vi "fakeScan.vi"() -> ()   [LabVIEW 2010]
uses:
  line_info.ctl
panel:
  out "line":T1
  out "size(s)":i32
  in  "CH1":bool=TRUE
  in  "CH0":bool=TRUE
  in  "xyz order":bool
  out "sort stats":T2
  out "assemble stats":T3
  in  "spilt ff/fb":bool
  out "lines":i32
  out "error out":errorcluster
  out "timed out?":bool
  out "XY view":T4(plugin-control)
  out "YZ view":T4(plugin-control)
  out "XZ view":T4(plugin-control)
  in  "scan specification":T5={"x amplitude"=100, "x resolution (pixels)"=30, "x offset fly-forward (iterations)"=57, "x offset fly-back (iterations)"=115, "y resolution (nr. of lines)"=79, "y step size"=41, "iterations per pixel"=5, "number of frames"=120, "y offset (pixels)"=0, "number of y-brake lines  (before y-fly-back)"=0, "number y-brake lines (after y-fly-back)"=30, "number of y-fly-back steps"=0, "lines per z step"=1, "number of z/intensity tuples"=342, "number of repetitions (volumes or planes)"=2, "z step size derived"=27, "choose the beginning of z scan"=FALSE, "number of frames (settings)"=120, "FPGA trajectory?"=TRUE, "Pockels cell voltage (bits)"=0, "Vy min(bits)"=-1638, "Vz min(bits)"=-1638}
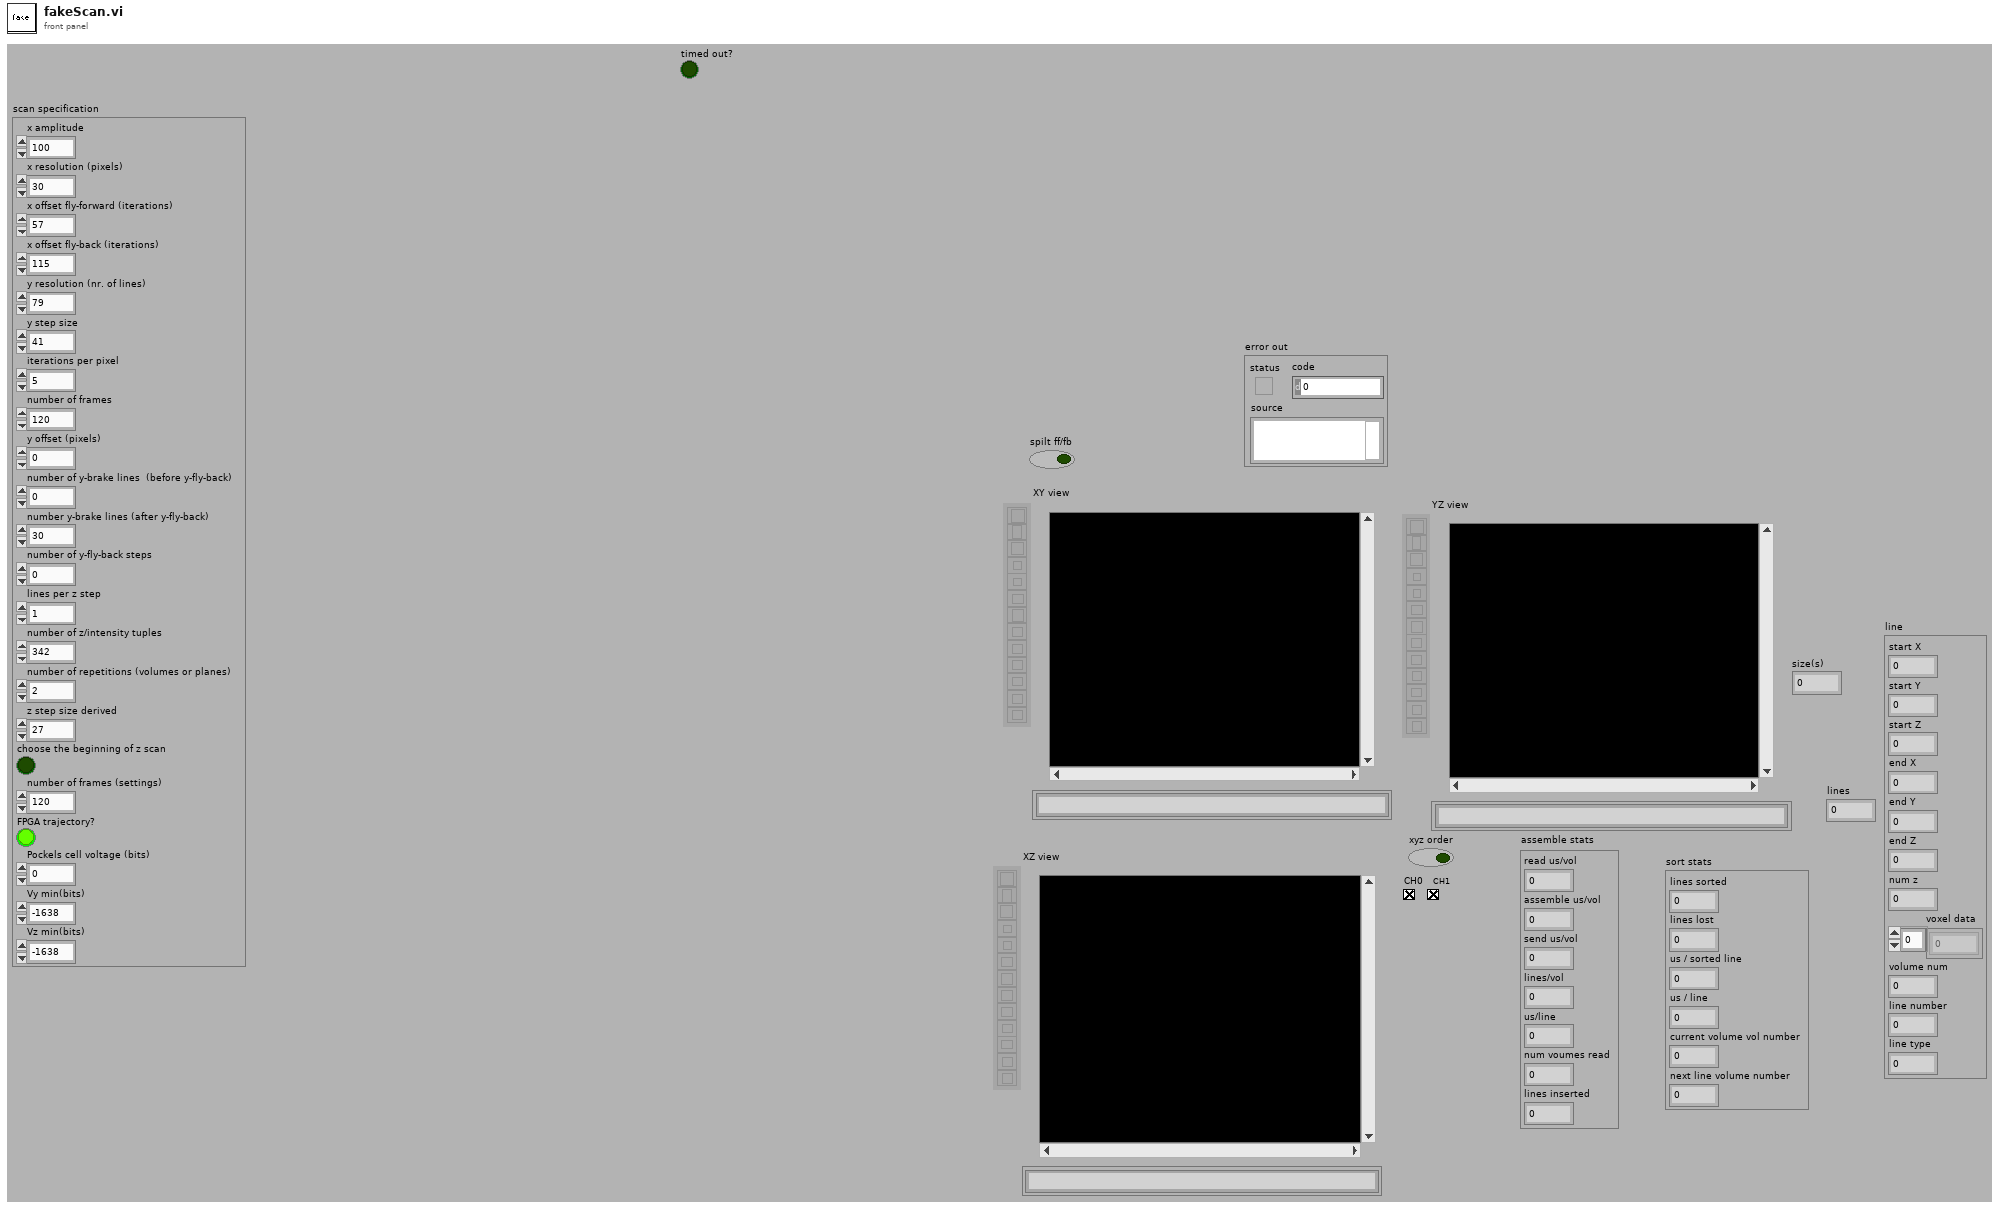
[diagram p1: front panel]
types:
  T1 = typedef "line_info.ctl" = cluster{"start X":i16, "start Y":i16, "start Z":i16, "end X":i16, "end Y":i16, "end Z":i16, "num z":u8, "voxel data":u32[], "volume num":u32, "line number":u16, "line type":u16}
  T2 = cluster{"lines sorted":i32, "lines lost":i32, "us / sorted line":dbl, "us / line":dbl, "current volume vol number":u32, "next line volume number":u32}
  T3 = cluster{"read us/vol":dbl, "assemble us/vol":dbl, "send us/vol":dbl, "lines/vol":dbl, "us/line":dbl, "num voumes read":u32, "lines inserted":i32}
  T4 = typedef "IMAQ Image.ctl" = refnum<image>
  T5 = cluster{"x amplitude":u16, "x resolution (pixels)":u16, "x offset fly-forward (iterations)":u16, "x offset fly-back (iterations)":u16, "y resolution (nr. of lines)":u16, "y step size":u16, "iterations per pixel":u16, "number of frames":i32, "y offset (pixels)":u16, "number of y-brake lines  (before y-fly-back)":u16, "number y-brake lines (after y-fly-back)":u16, "number of y-fly-back steps":u16, "lines per z step":u16, "number of z/intensity tuples":u16, "number of repetitions (volumes or planes)":i32, "z step size derived":u16, "choose the beginning of z scan":bool, "number of frames (settings)":i32, "FPGA trajectory?":bool, "Pockels cell voltage (bits)":i16, "Vy min(bits)":i16, "Vz min(bits)":i16}
  T6 = typedef "Image Type" = u32
  T7 = typedef "internal_queues.ctl" = cluster{"volumeQueue":refnum<queue>, "linesWithoutDataQueue":refnum<queue>, "lineQueue":refnum<queue>, "volumesWithLinesQueue":refnum<queue>, "kalmanQueue":refnum<queue>, "completedVolumeQueue":refnum<queue>, "displayVolumeQueue":refnum<queue>, "scanLocationsQueue":refnum<queue>, "kalmanToDisplayPanel":refnum<queue>, "focalPositionQueue":refnum<queue>, "spotPositionsToImagePanel":refnum<queue>}
  T8 = cluster{"min x":i16, "deltaX":dbl, "num x":u32, "max x":i16, "min y":i16, "deltaY":dbl, "num y":u32, "max y":i16, "num z":u32, "num voxels":u32, "voxels read":u32, "volume num":u32}
  T9 = cluster{"lines sorted":i32, "lines lost":i32, "us / sorted line":dbl, "us / line":dbl, "current volume vol number":u32, "next line volume number":u32, "volume rate(Hz)":dbl}
  T10 = cluster{"ch0 volume":u32[][][], "ch1 volume":u32[][][], "ff 0+1":u32[][][], "fb 0+1":u32[][][]}
  T11 = cluster{"New Image":T4, "New Image":T4, "New Image":T4}
  T12 = cluster{"Image Dst Out":T4, "Image Dst Out":T4, "Image Dst Out":T4}
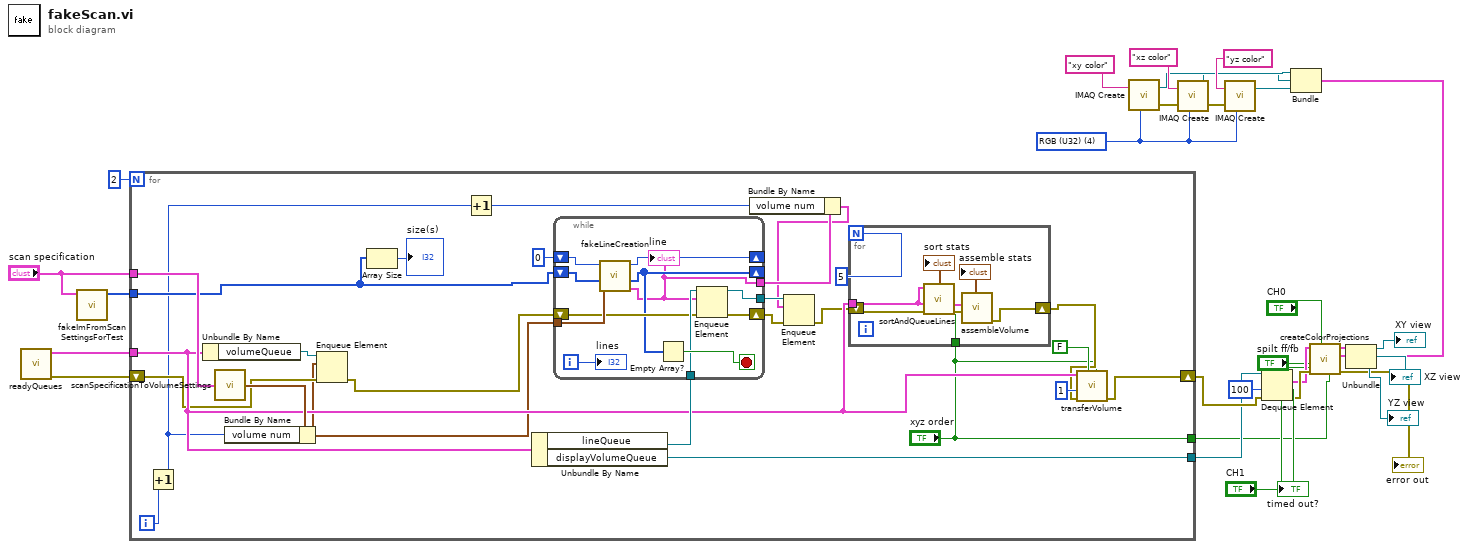
[diagram p0: block diagram]
diagram:
  w17 = T6 4 items=["Grayscale (U8)", "Grayscale (I16)", "Grayscale (SGL)", "Complex (CSG)", "RGB (U32)", "HSL (U32)", "RGB (U64)", "Grayscale (U16)"] ("Image Type")
  n1 = call "readyQueues.vi"() -> ("error out"=w8:errorcluster, "Queues"=w30:T7)  [unwired: 10 in]
  n2 = call "fakeImFromScanSettingsForTest.vi"("scan specification"="scan specification") -> ("fake 2 ch im"=w5:u32[])  [unwired: 10 in]
  n3 = for {
    N: 2 -> [_]
    tunnel: "scan specification" -> [w56]
    tunnel: w30 -> [w51]
    tunnel: [w47] -> w14
    shift-right: [w48] -> w15
    shift-left: w8 -> [w45]
    tunnel: w5 -> [w40]
    tunnel: ["xyz order"] -> w1
    i -> [w42]
    n4 = Increment(x=w42) -> (x+1=w33:i32)
    n5 = Unbundle By Name(w51) -> ("volumeQueue"=w36:refnum<queue>)
    n6 = call "scanSpecificationToVolumeSettings.vi"("scan specification"=w56) -> ("volume info"=w55:T8)
    n7 = Bundle By Name(cluster=w55, "volume num"=w33) -> (w43:T8)
    n8 = Enqueue Element(queue=w36, element=w43, error in (no error)=w45) -> (error out=w44:errorcluster)  [unwired: 1 in, 2 out]
    n9 = Array Size(array=w40) -> (size(s)=→"size(s)":i32)
    n10 = Increment(x=w33) -> (x+1=w32:i32)
    n11 = Unbundle By Name(w51) -> ("lineQueue"=w53:refnum<queue>, "displayVolumeQueue"=w47:refnum<queue>)
    n12 = while {
      tunnel: w43 -> [w75]
      shift-right: [w66] -> _
      shift-left: w40 -> [w67]
      shift-right: [w73] -> _
      shift-left: u32 0 ("voxel number out") -> [w72]
      tunnel: w53 -> [w71]
      shift-right: [w70] -> w38
      shift-left: w44 -> [w69]
      tunnel: [w65] -> w34
      tunnel: [w64] -> w35
      i -> [w68]
      stop <- w74 stop-if-true
      n13 = call "fakeLineCreation.vi"("volume info"=w75, "data stream in"=w67, "voxel number"=w72) -> ("line"=w65:T1, "data stream out"=w66:u32[], "voxel number out"=w73:u32)  [unwired: 6 in]
      "line" <- w65
      n14 = Empty Array?(array=w66) -> (empty?=w74:bool)
      n15 = Enqueue Element(queue=w71, element=w65, error in (no error)=w69) -> (queue out=w64:refnum<queue>, error out=w70:errorcluster)  [unwired: 1 in, 1 out]
      "lines" <- w68
    }
    n16 = Bundle By Name(cluster=w34, "volume num"=w32) -> (w31:T1)
    n17 = Enqueue Element(queue=w35, element=w31, error in (no error)=w38) -> (error out=w37:errorcluster)  [unwired: 1 in, 2 out]
    n18 = for {
      N: 5 -> [_]
      tunnel: w51 -> [w59]
      shift-right: [w63] -> w49
      shift-left: w37 -> [w61]
      tunnel: "xyz order" -> [w57]
      n19 = call "sortAndQueueLines.vi"("error in (no error)"=w61, "Queues"=w59) -> ("error out"=w60:errorcluster, "stats"=→"sort stats":T9)  [unwired: 6 in, 2 out]
      n20 = call "assembleVolume.vi"("error in (no error)"=w60, "xyz order"=w57, "Queues"=w59) -> ("error out"=w63:errorcluster, "status"=→"assemble stats":T3)  [unwired: 6 in, 1 out]
    }
    n21 = call "transferVolume.vi"("xyz order"="xyz order", "write to network stream"=FALSE, "error in (no error)"=w49, "num vol to sum"=u32 1, "Queues"=w51) -> ("error out"=w48:errorcluster)  [unwired: 1 in, 5 out]
  }
  n22 = call "IMAQ Create"("Image Name"="xy color", "Image Type"=w17) -> ("New Image"=w20:T4, "error out"=w22:errorcluster)  [unwired: 3 in]
  n23 = call "IMAQ Create"("Image Name"="xz color", "Image Type"=w17, "error in (no error)"=w22) -> ("New Image"=w19:T4, "error out"=w21:errorcluster)  [unwired: 2 in]
  n24 = call "IMAQ Create"("Image Name"="yz color", "Image Type"=w17, "error in (no error)"=w21) -> ("New Image"=w18:T4)  [unwired: 2 in, 1 out]
  n25 = Dequeue Element(queue=w14, timeout in ms (-1)=100, error in (no error)=w15) -> (element=w10:T10, timed out?=→"timed out?":bool, error out=w11:errorcluster)  [unwired: 1 out]
  n26 = Bundle("New Image"=w20, "New Image"=w19, "New Image"=w18) -> (w16:T11)  [unwired: 1 in]
  n27 = call "createColorProjections.vi"("xyz order"=w1, "max values"="CH1", "display channels"="CH0", "error in (no error)"=w11, "spilt ff/fb"="spilt ff/fb", "color ims"=w16, "volumes for display"=w10) -> ("error out"=→"error out":errorcluster, "color ims out"=w29:T12)  [unwired: 3 out]
  n28 = Unbundle(w29) -> ("Image Dst Out"=→"XY view":T4, "Image Dst Out"=→"XZ view":T4, "Image Dst Out"=→"YZ view":T4)
